vi "Fresh Water Calinration.vi"(11 "Sample Size for Density Meter Reading  in":i32=20) -> (2 "Fresh Reading Fill Density Meter":dbl, 3 "Fresh Reading Portable Density Meter":dbl format="%.2f")   [LabVIEW 2011]
uses:
  ADAM Client/Sub VIs/ADAM Controls/Address.ctl
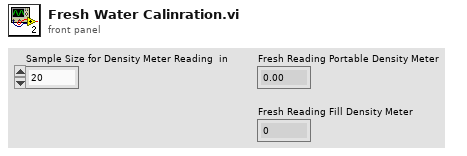
[diagram p1: front panel]
types:
  T1 = typedef "Address.ctl" = cluster{"Main":i32, "Ch.":i32, "Sub":i32, "Port Name":string}
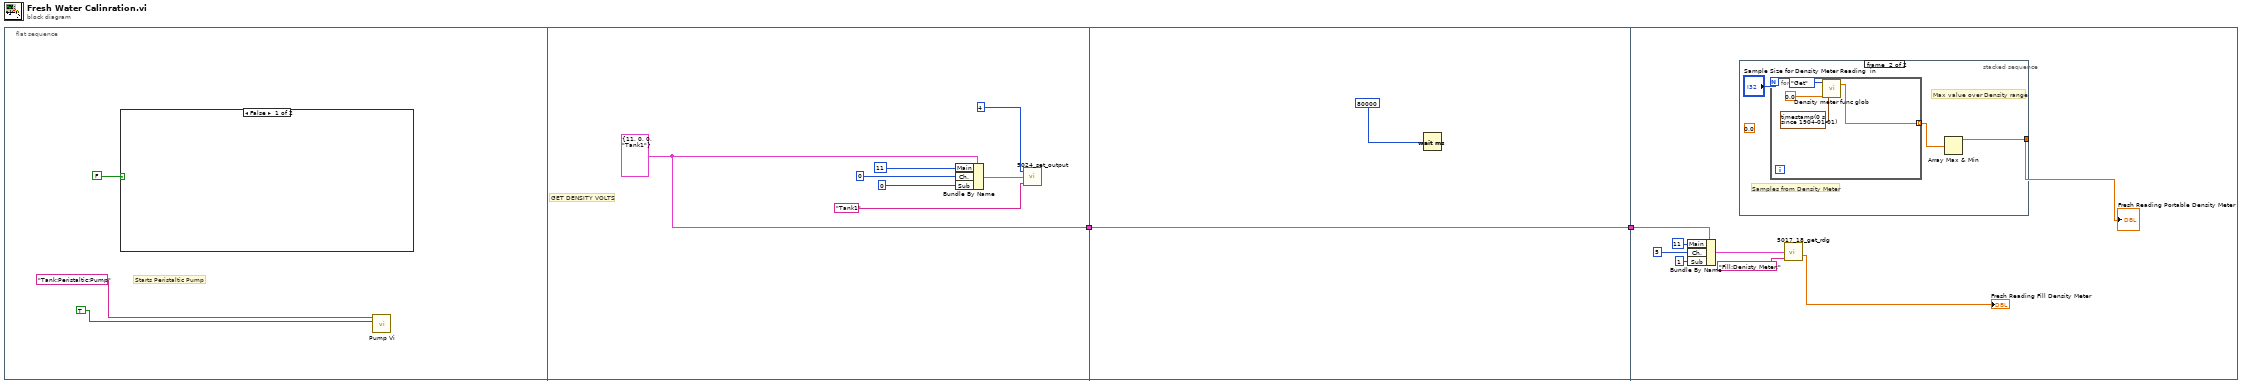
[diagram p0: block diagram]
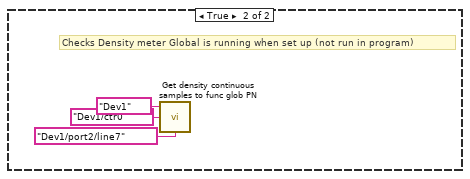
[diagram p2: hidden frame]
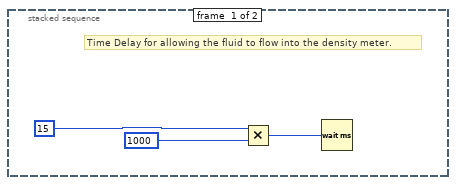
[diagram p3: hidden frame]
diagram:
  n1 = flat-sequence {
    tunnel: [w9] -> w2
    tunnel: [w16] -> w1
    tunnel: w2 -> [w16]
    tunnel: w1 -> [w18]
    frame #0 {
      # "Starts Peristaltic Pump"
      n2 = case shown="False" FALSE {
        frame False {
        }
        frame True {
          # "Checks Density meter Global is running when set up (not run in program)"
          n3 = call "Get density continuous samples to func glob PN.vi"("Timing SW trigger"=tag "Dev1/port2/line7", "Counter"=tag "Dev1/ctr0", "Device"=tag "Dev1") -> ()
        }
      }
      n4 = call "Pump Vi.vi"("Boolean"=TRUE, "Channel Name"="Tank:Peristaltic:Pump") -> ()  [unwired: 8 in, 2 out]
    }
    frame #1 {
      w9 = T1 {"Main"=11, "Ch."=0, "Sub"=0, "Port Name"="Tank1"} ("Address (all reqd.)")
      # "GET DENSITY VOLTS"
      n5 = Bundle By Name(cluster=w9, "Main"=11, "Ch."=0, "Sub"=0) -> (w11:T1)
      n6 = call "5024_set_output.vi"("Set to:"=4, "Address (all reqd.)"=w11, "Channel Name"="Tank1" ("Port Name")) -> ()  [unwired: 2 in, 2 out]
    }
    frame #2 {
      n7 = Wait (ms)(milliseconds to wait=80000) -> ()  [unwired: 1 out]
    }
    frame #3 {
      n8 = Bundle By Name(cluster=w18, "Main"=11, "Ch."=5, "Sub"=1) -> (w23:T1)
      n9 = stacked-sequence {
        tunnel: [_ w30] -> w25
        frame #0 {
          # "Time Delay for allowing the fluid to flow into the density meter."
          n10 = Multiply(x=15 ("Sample Size 2"), y=1000 ("Sample Size 2")) -> (x*y=w27:i32)
          n11 = Wait (ms)(milliseconds to wait=w27) -> ()  [unwired: 1 out]
        }
        frame #1 {
          (unwired) 0.0 ("Actual Density (kg/m3) 2")
          # "Max value over Density range"
          # "Samples from Density Meter"
          n12 = for {
            N: "Sample Size for Density Meter Reading  in" -> [_]
            tunnel: [w32] -> w29 mode=indexing
            n13 = call "Density meter func glob.vi"("Sample DateTime in"=timestamp(0 s since 1904-01-01), "Density in"=0.0, "Action"=enum16{"Get", "Set"}."Get") -> ("Density out"=w32:dbl)  [unwired: 1 out]
          }
          n14 = Array Max & Min(array=w29) -> (max value=w30:dbl)  [unwired: 3 out]
        }
      }
      "Fresh Reading Portable Density Meter" <- w25
      n15 = call "5017_18_get_rdg.vi"("Address (all reqd.)"=w23, "Channel Name"="Fill:Denisty Meter:") -> ("Reading"=→"Fresh Reading Fill Density Meter":dbl)  [unwired: 3 in, 1 out]
    }
  }
